vi "初始化.vi"(8 "error in (no error)":errorcluster caption="错误输入（无错误）", 9 "设定时间":u32[](array[numeric]), 11 "信号灯成员类 输入":refnum<class "信号灯成员类.lvclass">) -> (0 "error out":errorcluster caption="错误输出", 3 "信号灯成员类 输出":refnum<class "信号灯成员类.lvclass">)   [LabVIEW 2017, in "信号灯成员类.lvclass"]
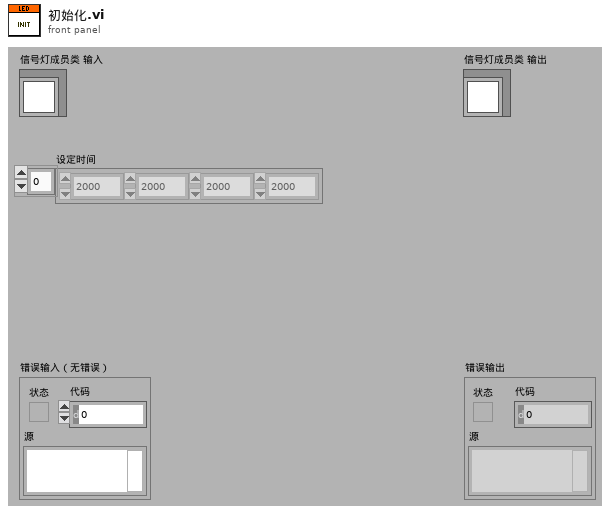
[diagram p1: front panel]
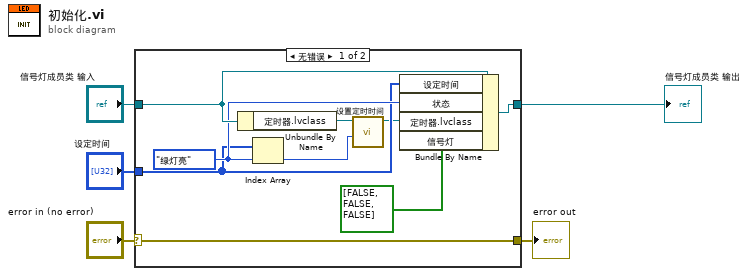
[diagram p0: block diagram]
diagram:
  n1 = case shown="无错误" "error in (no error)" {
    selector: "error in (no error)" -> [w14 w16]
    tunnel: [w14 w16] -> w4
    tunnel: [w13 w15] -> w2
    tunnel: "信号灯成员类 输入" -> [w12 w15]
    tunnel: "设定时间" -> [w9 _]
    frame No Error {
      w10 = enum16{"绿灯亮", "黄灯亮", "红灯亮", "全部亮", "全部熄灭"}."绿灯亮" ("状态")
      n2 = Unbundle By Name(w12) -> ("定时器.lvclass"=w11:refnum<class "定时器.lvclass">)
      n3 = Index Array(array=w9, index=w10) -> (element=w8:u32)
      n4 = call-dynamic "设置定时时间.vi"("设置时间"=w8, "定时器 输入"=w11) -> ("定时器 输出"=w7:refnum<class "定时器.lvclass">)  [unwired: 1 in, 8 out]
      n5 = Bundle By Name(cluster=w12, "设定时间"=w9, "状态"=w10, "定时器.lvclass"=w7, "信号灯"=bool[] [FALSE, FALSE, FALSE]) -> (w13:refnum<class "信号灯成员类.lvclass">)
    }
    frame Error {
    }
  }
  "error out" <- w4
  "信号灯成员类 输出" <- w2
